vi "Append error.vi"(8 "error in (no error)":errorcluster, 9 "error":errorcluster, 11 "Simulated_CCD_Camera in":refnum<class "Simulated Camera.lvclass">) -> (0 "error out":errorcluster, 3 "Simulated_CCD_Camera out":refnum<class "Simulated Camera.lvclass">)   [LabVIEW 2018, in "Simulated Camera.lvclass"]
doc: "Append an error to the array of errors of the class\n\nThis array is verified before the start of an exposure. If an error is found, the exposure will not occur."
uses:
  Simulated Camera.lvclass
  Simulated Camera.lvclass/Simulated Camera.ctl
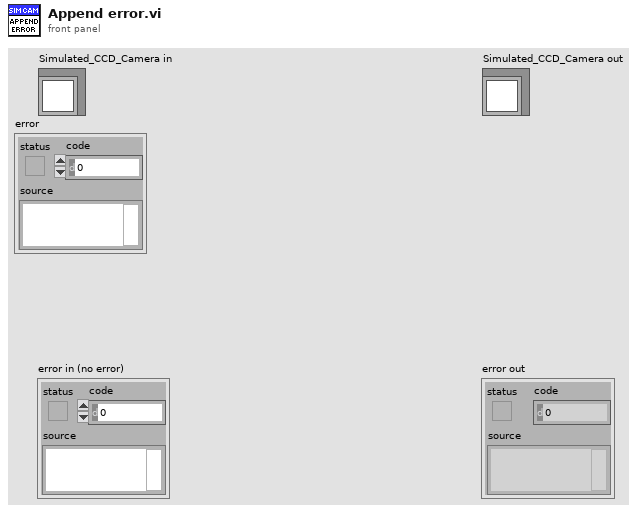
[diagram p1: front panel]
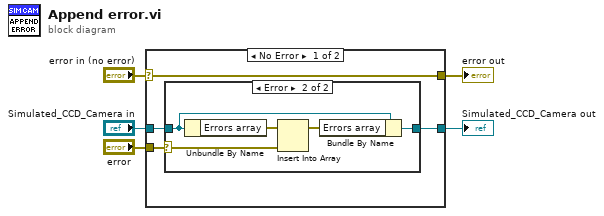
[diagram p0: block diagram]
diagram:
  n1 = case shown="No Error" "error in (no error)" {
    selector: "error in (no error)" -> [w9 w17]
    tunnel: [w9 w17] -> w4
    tunnel: [w7 w16] -> w2
    tunnel: "Simulated_CCD_Camera in" -> [w8 w16]
    tunnel: "error" -> [w6 _]
    frame No Error {
      n2 = case shown="Error" w6 {
        selector: w6 -> [_ w11]
        tunnel: w8 -> [w10 w14]
        tunnel: [w10 w13] -> w7
        frame No Error {
        }
        frame Error {
          n3 = Unbundle By Name(w14) -> ("Errors array"=w15:errorcluster[])
          n4 = Insert Into Array(array=w15, new element=w11) -> (w12:errorcluster[])  [unwired: 1 in]
          n5 = Bundle By Name(cluster=w14, "Errors array"=w12) -> (w13:refnum<class "Simulated Camera.lvclass">)
        }
      }
    }
    frame Error {
    }
  }
  "error out" <- w4
  "Simulated_CCD_Camera out" <- w2
